vi "系统设置_其他.vi"() -> ()   [LabVIEW 2016]
uses:
  <vilib>/Utility/sysdir.llb/System Directory Type.ctl
  <vilib>/Utility/miscctls.llb/LVPointTypeDef.ctl
  <vilib>/addons/database/Connection.llb/DB Tools Open Connec (String).vi
  <vilib>/addons/database/NI_Database_API.lvlib
panel:
  in  "布尔":bool
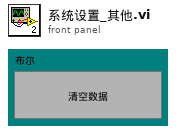
[diagram p1: front panel]
types:
  T1 = typedef "System Directory Type.ctl" = i32
  T2 = typedef "NI_Database_API.lvlib/Conn ObjectReference.ctl" = refnum<k1>
  T3 = typedef "LVPointTypeDef.ctl" = cluster{"Horizontal":i16, "Vertical":i16}
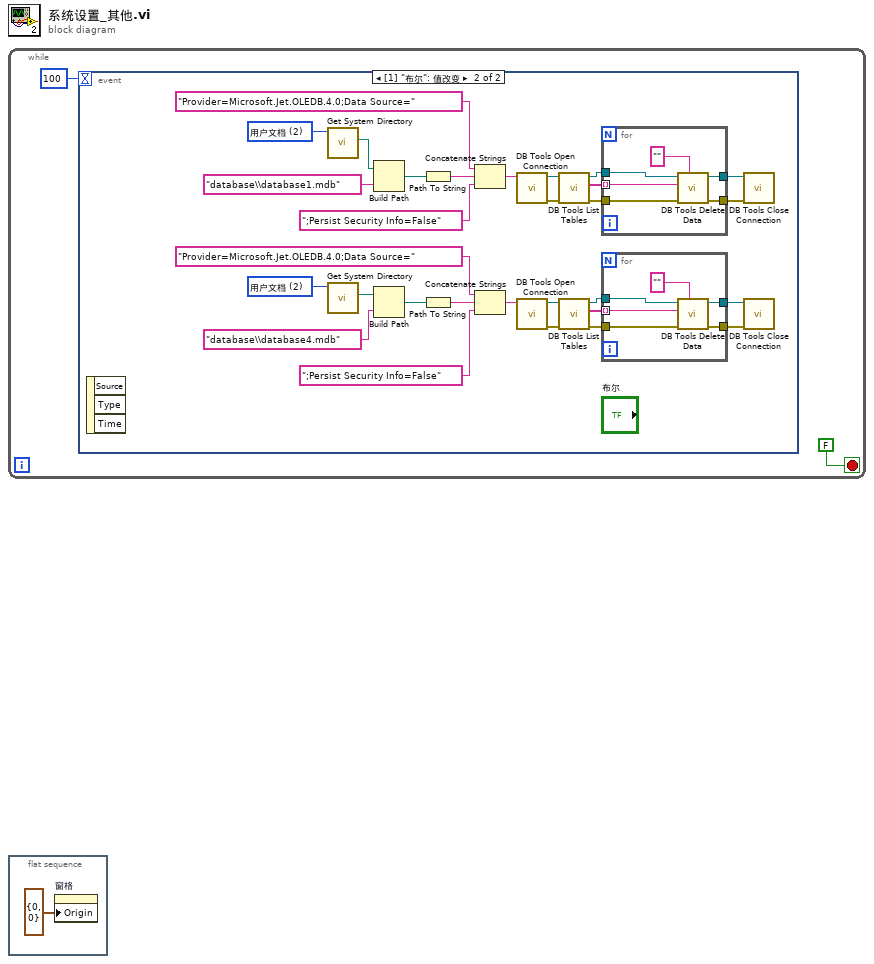
[diagram p0: block diagram]
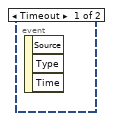
[diagram p2: hidden frame]
diagram:
  n1 = while {
    stop <- FALSE stop-if-true
    n2 = event shown="[1] \"布尔\": 值改变" {
      selector: _ -> [_ _]
      dyn-events: _ -> [_ _]
      timeout: 100 -> [_ _]
      event Timeout {
        n3 = event-data() -> ()  [unwired: 1 in, 3 out]
      }
      event "布尔": Value Change {
        w28 = T1 2 items=["用户目录"=0, "用户桌面"=1, "用户文档"=2, "用户应用程序数据"=3, "用户设置"=4, "用户临时目录"=5, "公共文档"=6, "公共应用程序数据"=7, "公共设置"=8, "公共缓存"=13, "系统核心库"=9, "系统安装库"=10, "应用程序文件"=11, "启动盘根目录"=12] ("system directory type")
        w7 = T1 2 items=["用户目录"=0, "用户桌面"=1, "用户文档"=2, "用户应用程序数据"=3, "用户设置"=4, "用户临时目录"=5, "公共文档"=6, "公共应用程序数据"=7, "公共设置"=8, "公共缓存"=13, "系统核心库"=9, "系统安装库"=10, "应用程序文件"=11, "启动盘根目录"=12] ("system directory type")
        n4 = event-data() -> ()  [unwired: 1 in, 3 out]
        n5 = call <vilib>:"Get System Directory.vi"("system directory type"=w28) -> ("system directory"=w27:path)  [unwired: 10 in]
        n6 = call <vilib>:"Get System Directory.vi"("system directory type"=w7) -> ("system directory"=w8:path)  [unwired: 10 in]
        n7 = Build Path(base path=w27, name or relative path="database\\database1.mdb" ("名称或相对路径")) -> (appended path=w29:path)
        n8 = Build Path(base path=w8, name or relative path="database\\database4.mdb" ("名称或相对路径")) -> (appended path=w6:path)
        n9 = Path To String(path=w29) -> (string=w30:string)
        n10 = Path To String(path=w6) -> (string=w5:string)
        n11 = Concatenate Strings("Provider=Microsoft.Jet.OLEDB.4.0;Data Source=", w30, ";Persist Security Info=False") -> (w25:string)
        n12 = Concatenate Strings("Provider=Microsoft.Jet.OLEDB.4.0;Data Source=", w5, ";Persist Security Info=False") -> (w10:string)
        n13 = call-poly <vilib>:"DB Tools Open Connection.vi"("connection information"=w25) -> ("error out"=w23:errorcluster, "connection reference"=w24:T2)  [unwired: 7 in]
        n14 = call-poly <vilib>:"DB Tools Open Connection.vi"("connection information"=w10) -> ("error out"=w12:errorcluster, "connection reference"=w11:T2)  [unwired: 7 in]
        n15 = call <vilib>:"DB Tools List Tables.vi"("error in (no error)"=w23, "connection reference"=w24) -> ("error out"=w20:errorcluster, "tables"=w22:string[], "connection reference out"=w21:T2)  [unwired: 3 in]
        n16 = call <vilib>:"DB Tools List Tables.vi"("error in (no error)"=w12, "connection reference"=w11) -> ("error out"=w15:errorcluster, "tables"=w13:string[], "connection reference out"=w14:T2)  [unwired: 3 in]
        n17 = for {
          tunnel: w22 -> [w36] mode=indexing
          tunnel: w21 -> [w38]
          tunnel: w20 -> [w37]
          tunnel: [w34] -> w19
          tunnel: [w33] -> w18
          n18 = call <vilib>:"DB Tools Delete Data.vi"("condition"="", "error in (no error)"=w37, "table"=w36, "connection reference"=w38) -> ("error out"=w33:errorcluster, "connection reference out"=w34:T2)  [unwired: 6 in]
        }
        n19 = for {
          tunnel: w13 -> [w42] mode=indexing
          tunnel: w14 -> [w44]
          tunnel: w15 -> [w43]
          tunnel: [w40] -> w16
          tunnel: [w39] -> w17
          n20 = call <vilib>:"DB Tools Delete Data.vi"("condition"="", "error in (no error)"=w43, "table"=w42, "connection reference"=w44) -> ("error out"=w39:errorcluster, "connection reference out"=w40:T2)  [unwired: 6 in]
        }
        n21 = call <vilib>:"DB Tools Close Connection.vi"("error in (no error)"=w18, "connection reference"=w19) -> ()  [unwired: 5 in, 1 out]
        n22 = call <vilib>:"DB Tools Close Connection.vi"("error in (no error)"=w17, "connection reference"=w16) -> ()  [unwired: 5 in, 1 out]
      }
    }
  }
  n23 = flat-sequence {
    frame #0 {
      n24 = property on="窗格" class="Pane"("Origin"=T3 {"Horizontal"=0, "Vertical"=0} ("原点")) -> ()  [unwired: 2 in, 2 out]
    }
  }
